vi "Set SubPanel.vi"(8 "error in (no error)":errorcluster, 10 "SubPanel":refnum<vi>, 11 "Panel in":refnum<class "Panel.lvclass">) -> (0 "error out":errorcluster, 3 "Panel out":refnum<class "Panel.lvclass">)   [LabVIEW 2020, in "OOPanel.lvlib" / "Panel.lvclass"]
uses:
  Panel.lvclass
  Panel.lvclass/Panel.ctl
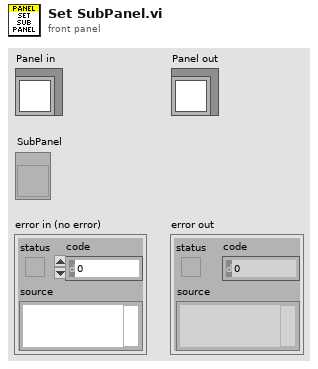
[diagram p1: front panel]
types:
  T1 = typedef "OOPanel.lvlib/Panel.lvclass/Ref Data.ctl" = cluster{"Panel Events":T2, "Panel Ref":refnum<vi>, "SubPanel":refnum<vi>, "Close":bool, "Running":bool, "State":T3}
  T2 = typedef "OOPanel.lvlib/Panel.lvclass/Panel Events.ctl" = cluster{"Visbility":refnum<user-event>, "Close":refnum<user-event>}
  T3 = typedef "OOPanel.lvlib/Panel.lvclass/Visibility State.ctl" = enum16{"Idle", "Closed", "Hidden", "Visible", "Subpanel"}
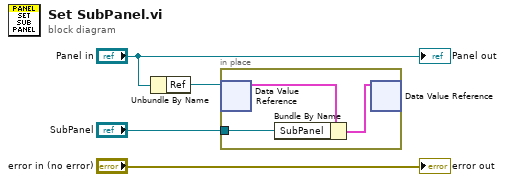
[diagram p0: block diagram]
diagram:
  n1 = Unbundle By Name("Panel in") -> ("Ref"=w3:refnum<data-value>)
  n2 = in-place {
    in-place-border: "SubPanel" -> [w5]
    n3 = in-place-dvr #1(w3) -> (w7:T1)  [unwired: 1 out]
    n4 = Bundle By Name(cluster=w7, "SubPanel"=w5) -> (w6:T1)
    n5 = in-place-dvr #1(w6) -> ()  [unwired: 2 out]
  }
  "error out" <- "error in (no error)"
  "Panel out" <- "Panel in"
